vi "FFT.vi"() -> ()   [LabVIEW 2015]
uses:
  <vilib>/vision/NI_Vision_Development_Module.lvlib
panel:
  in  "percent":dbl(slide) scale=0.0..100.0
  in  "index":u8(slide) scale=-1.0..121.0
  out "Filtered FFT":T1(plugin-control)
  out "Mask":T1(plugin-control)
  out "FFT":T1(plugin-control)
  out "Source":T1(plugin-control)
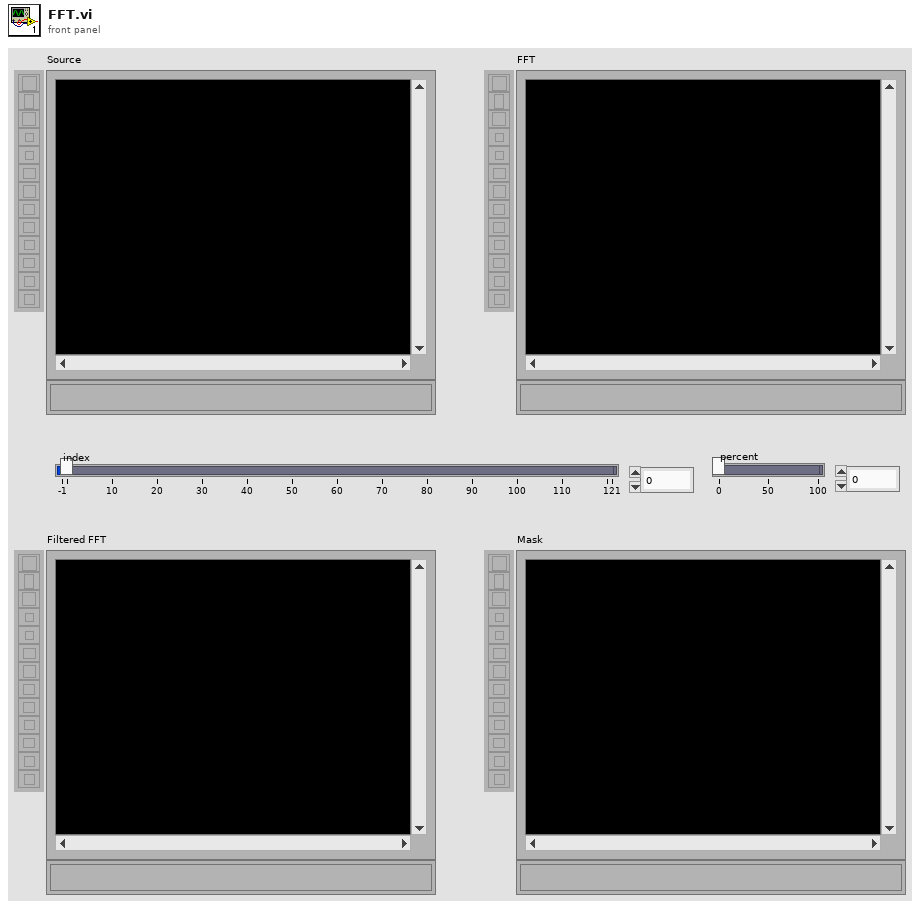
[diagram p1: front panel]
types:
  T1 = typedef "IMAQ Image.ctl" = refnum<image>
  T2 = typedef "Image Type" = u32
  T3 = typedef "ROI Descriptor" = cluster{"Global Rectangle":i32[], "Contours":cluster{"ID":enum32{"External", "Internal"}, "Type":u32, "Coordinates":i32[]}[]}
  T4 = cluster{"ID":enum32{"External", "Internal"}, "Type":i32, "Coordinates":i32[]}
  T5 = cluster{"ID":enum32{"External", "Internal"}, "Type":i32, "Coordinates":i32[]}[]
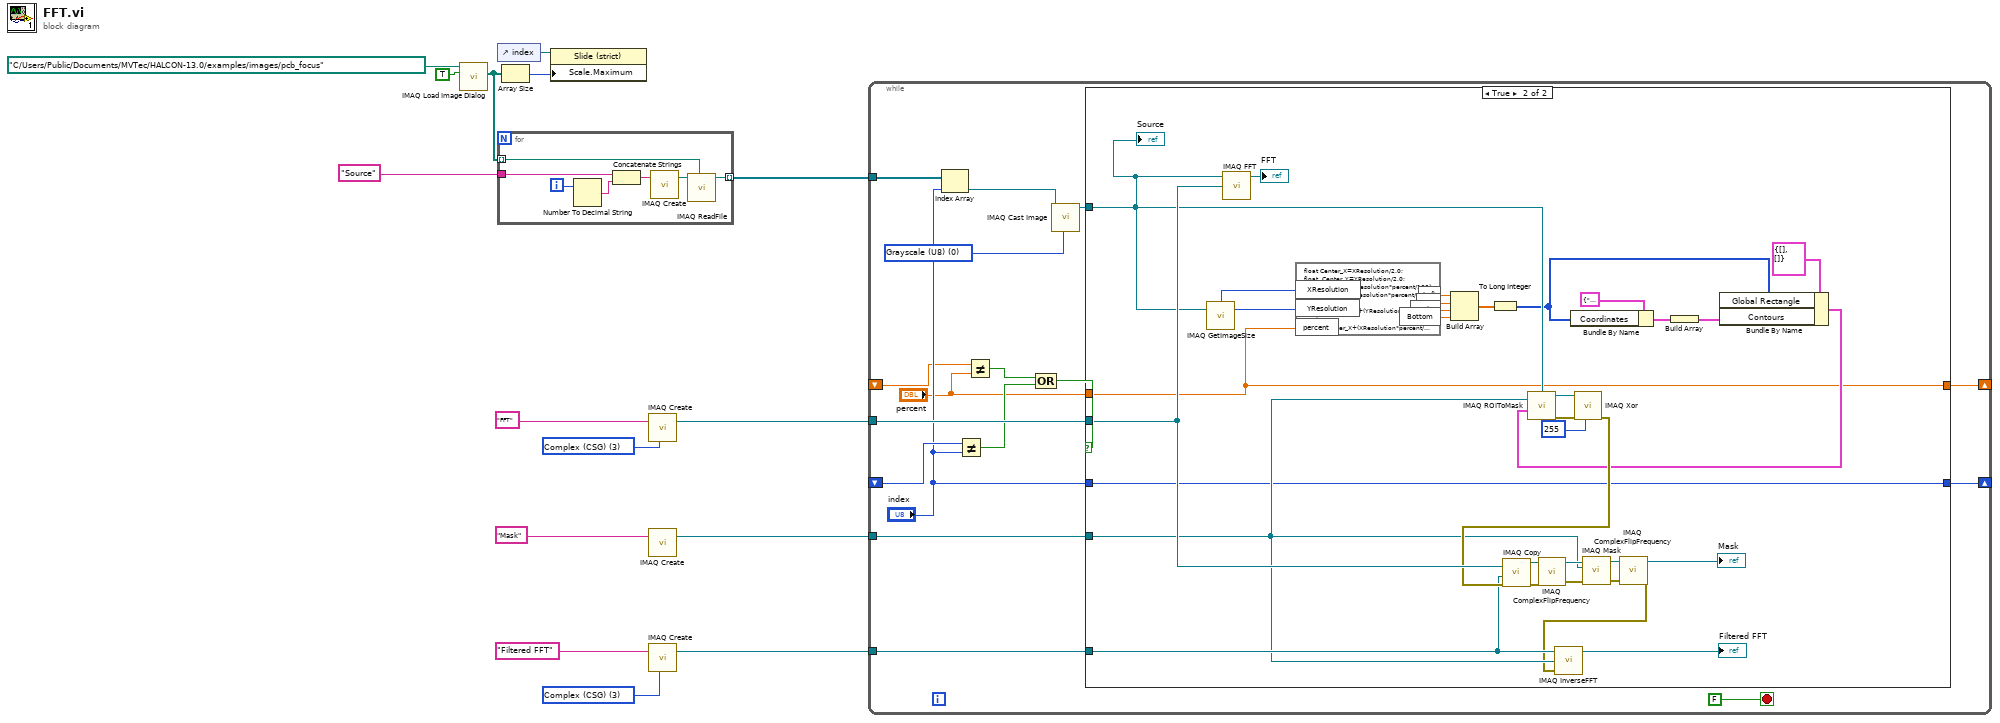
[diagram p0: block diagram]
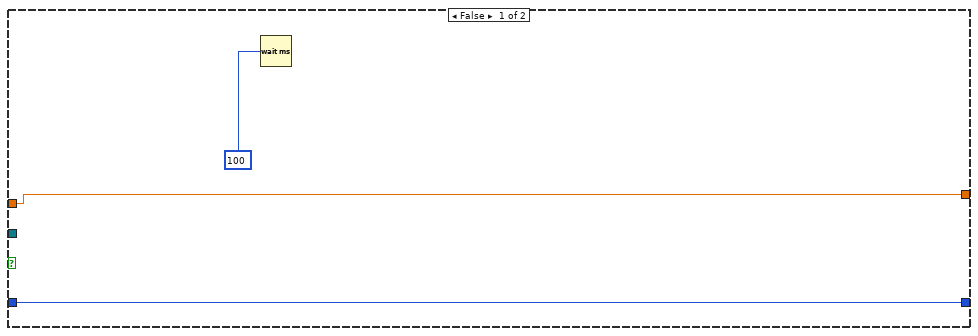
[diagram p2: hidden frame]
diagram:
  w13 = T2 3 items=["Grayscale (U8)", "Grayscale (I16)", "Grayscale (SGL)", "Complex (CSG)", "RGB (U32)", "HSL (U32)", "RGB (U64)", "Grayscale (U16)"] ("Image Type")
  w14 = T2 3 items=["Grayscale (U8)", "Grayscale (I16)", "Grayscale (SGL)", "Complex (CSG)", "RGB (U32)", "HSL (U32)", "RGB (U64)", "Grayscale (U16)"] ("Image Type")
  n1 = call "IMAQ Load Image Dialog"("Multiple Files? (No)"=TRUE, "Start Path"=path "C:/Users/Public/Documents/MVTec/HALCON-13.0/examples/images/pcb_focus") -> ("Paths"=w4:path[])  [unwired: 7 in, 2 out]
  n2 = control-ref of="index"() -> (w5:refnum<vi>)
  n3 = for {
    tunnel: w4 -> [w22] mode=indexing
    tunnel: "Source" ("Image Name") -> [w19]
    tunnel: [w16] -> w2 mode=indexing
    i -> [w20]
    n4 = Number To Decimal String(number=w20) -> (decimal integer string=w18:string)  [unwired: 1 in]
    n5 = Concatenate Strings(w19, w18) -> (w17:string)
    n6 = call "IMAQ Create"("Image Name"=w17) -> ("New Image"=w21:T1)  [unwired: 4 in, 1 out]
    n7 = call "IMAQ ReadFile"("File Path"=w22, "Image"=w21) -> ("Image Out"=w16:T1)  [unwired: 5 in, 4 out]
  }
  n8 = Array Size(array=w4) -> (size(s)=w3:i32)
  n9 = property class="Slide (strict)"(reference=w5, "Scale.Maximum"=w3) -> ()  [unwired: 1 in, 2 out]
  n10 = call "IMAQ Create"("Image Name"="FFT", "Image Type"=w14) -> ("New Image"=w10:T1)  [unwired: 3 in, 1 out]
  n11 = call "IMAQ Create"("Image Name"="Mask") -> ("New Image"=w8:T1)  [unwired: 4 in, 1 out]
  n12 = call "IMAQ Create"("Image Name"="Filtered FFT", "Image Type"=w13) -> ("New Image"=w9:T1)  [unwired: 3 in, 1 out]
  n13 = while {
    tunnel: w10 -> [w39]
    tunnel: w9 -> [w38]
    tunnel: w8 -> [w37]
    tunnel: w2 -> [w35]
    shift-right: [w32] -> _
    shift-left: _ -> [w34]
    shift-right: [w28] -> _
    shift-left: _ -> [w27]
    stop <- FALSE stop-if-true
    w30 = T2 0 items=["Grayscale (U8)", "Grayscale (I16)", "Grayscale (SGL)", "Complex (CSG)", "RGB (U32)", "HSL (U32)", "RGB (U64)", "Grayscale (U16)"] ("Image Type")
    n14 = Index Array(array=w35, index="index") -> (element=w31:T1)
    n15 = Not Equal?(x=w34, y="index") -> (x != y?=w25:bool)
    n16 = Not Equal?(x=w27, y="percent") -> (x != y?=w26:bool)
    n17 = Compound Arithmetic op=OR(w26, w25) -> (w24:bool)
    n18 = call "IMAQ Cast Image"("Image Type"=w30, "Image Src"=w31) -> ("Image Dst Out"=w29:T1)  [unwired: 8 in, 1 out]
    n19 = case shown="True" w24 {
      tunnel: w29 -> [_ w58]
      tunnel: w39 -> [_ w71]
      tunnel: w38 -> [_ w68]
      tunnel: w37 -> [_ w67]
      tunnel: "index" -> [w42 w59]
      tunnel: [w42 w59] -> w32
      tunnel: [w40 w45] -> w28
      tunnel: "percent" -> [w40 w45]
      frame False {
        n20 = Wait (ms)(milliseconds to wait=u32 100) -> ()  [unwired: 1 out]
      }
      frame True {
        n21 = call "IMAQ GetImageSize"("Image"=w58) -> ("Y Resolution"=w56:i32, "X Resolution"=w57:i32)  [unwired: 3 in, 1 out]
        n22 = call "IMAQ FFT"("Image Dst"=w71, "Image Src"=w58) -> ("Image Dst Out"=→"FFT":T1)  [unwired: 2 in, 1 out]
        n23 = formula code="float Center_X=XResolution/2.0;\nfloat  Center_Y=YResolution/2.0;\nTop=Center_Y-(YResolution*percent/100);\nLeft=Center_X-(XResolution*percent/100);\nBottom=Center_Y+(YResolution*percent/100);\nRight=Center_X+(XResolution*percent/100);"("XResolution"=w57, "YResolution"=w56, "percent"=w45) -> ("Left"=w52:dbl, "Top"=w53:dbl, "Right"=w54:dbl, "Bottom"=w55:dbl)
        n24 = Build Array(w52, w53, w54, w55) -> (w51:dbl[])
        n25 = To Long Integer(number=w51) -> (32bit integer=w49:i32[])
        n26 = Bundle By Name(cluster=T4 {"ID"=enum."External", "Type"=4, "Coordinates"=[]}, "Coordinates"=w49) -> (w48:T4)
        n27 = Build Array(w48) -> (w47:T5)
        n28 = Bundle By Name(cluster=T3 {"Global Rectangle"=[], "Contours"=[]} ("ROI Descriptor"), "Global Rectangle"=w49, "Contours"=w47) -> (w46:T3)
        n29 = call "IMAQ ROIToMask"("ROI Descriptor"=w46, "Image"=w67, "Image Model"=w58) -> ("error out"=w64:errorcluster, "Image Out"=w63:T1)  [unwired: 3 in, 1 out]
        n30 = call "IMAQ Xor"("Constant"=i64 255, "error in (no error)"=w64, "Image Src A"=w63) -> ("error out"=w69:errorcluster)  [unwired: 7 in, 1 out]
        n31 = call "IMAQ Copy"("error in (no error)"=w69, "Image Dst"=w68, "Image Src"=w71) -> ("error out"=w62:errorcluster, "Image Dst Out"=w74:T1)  [unwired: 3 in]
        n32 = call "IMAQ ComplexFlipFrequency"("error in (no error)"=w62, "Image Src"=w74) -> ("error out"=w61:errorcluster, "Image Dst Out"=w73:T1)  [unwired: 2 in]
        n33 = call "IMAQ Mask"("error in (no error)"=w61, "Image Mask"=w67, "Image Src"=w73) -> ("error out"=w60:errorcluster, "Image Dst Out"=w72:T1)  [unwired: 2 in]
        n34 = call "IMAQ ComplexFlipFrequency"("error in (no error)"=w60, "Image Src"=w72) -> ("error out"=w65:errorcluster, "Image Dst Out"=→"Mask":T1)  [unwired: 2 in]
        n35 = call "IMAQ InverseFFT"("error in (no error)"=w65, "Image Dst"=w67, "Image Src"=w68) -> ("Image Dst Out"=→"Filtered FFT":T1)  [unwired: 1 in, 1 out]
        "Source" <- w58
      }
    }
  }
